vi "Add Message Handler.vi"(8 "error in (no error)":errorcluster, 10 "TCPMessageHandler":refnum<class "TCPMessageHandler.lvclass">, 11 "TCPMessageAPI in":refnum<class "TCPMessageAPI.lvclass">) -> (0 "error out":errorcluster, 3 "TCPMessageAPI out":refnum<class "TCPMessageAPI.lvclass">)   [LabVIEW 2020, in "Vecto.lvlib" / "TCPMessageAPI.lvclass"]
uses:
  TCPMessageAPI.lvclass
  TCPMessageHandler/TCPMessageHandler.lvclass
  TCPMessageAPI.lvclass/TCPMessageAPI.ctl
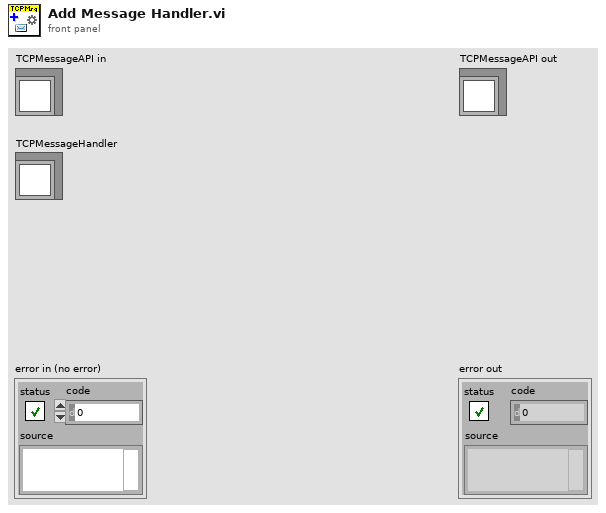
[diagram p1: front panel]
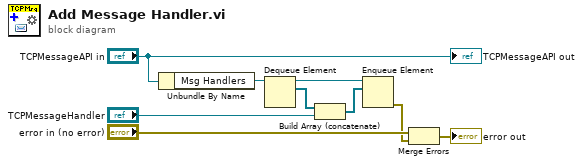
[diagram p0: block diagram]
diagram:
  n1 = Unbundle By Name("TCPMessageAPI in") -> ("Msg Handlers"=w7:refnum<queue>)
  n2 = Dequeue Element(queue=w7) -> (queue out=w4:refnum<queue>, element=w5:refnum<class "TCPMessageHandler.lvclass">[])  [unwired: 2 in, 2 out]
  n3 = Build Array (concatenate)(w5, "TCPMessageHandler") -> (w3:refnum<class "TCPMessageHandler.lvclass">[])
  n4 = Enqueue Element(queue=w4, element=w3) -> (error out=w1:errorcluster)  [unwired: 2 in, 2 out]
  n5 = Merge Errors("error in (no error)", w1) -> (→"error out":errorcluster)
  "TCPMessageAPI out" <- "TCPMessageAPI in"
